vi "DrawGoal.vi"(8 "error in (no error)":errorcluster, 10 "point":cluster{"x":dbl, "y":dbl}, 11 "picture":picture) -> (0 "error out":errorcluster, 3 "new picture":picture)   [LabVIEW 2009, in "Host.lvlib" / "Draw.lvlib"]
uses:
  Draw.lvlib
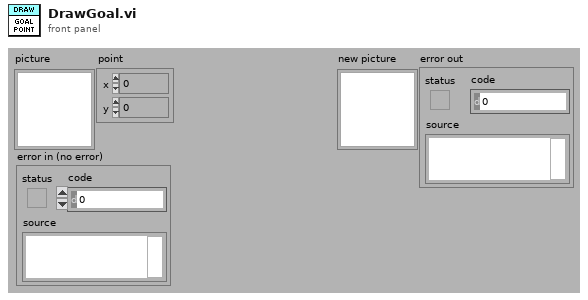
[diagram p1: front panel]
types:
  T1 = cluster{"Width":u16, "Style":enum32{"Solid", "Dash", "Dot", "DashDot", "DashDotDot"}}
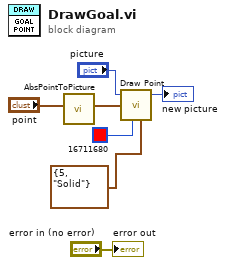
[diagram p0: block diagram]
diagram:
  n1 = call "AbsPointToPicture.vi"("input position"="point") -> ("output point"=w1:cluster{"x":i16, "y":i16})  [unwired: 10 in]
  n2 = call <vilib>:"Draw Point.vi"("picture"="picture", "point(x,y)"=w1, "color(black)"=u32 16711680, "pen"=T1 {"Width"=5, "Style"=enum."Solid"}) -> ("new picture"=→"new picture":picture)  [unwired: 5 in]
  "error out" <- "error in (no error)"
